vi "state.vi"(1 "buffer in":string) -> (0 "current state":dbl)   [LabVIEW 2016]
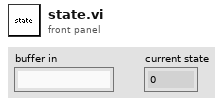
[diagram p1: front panel]
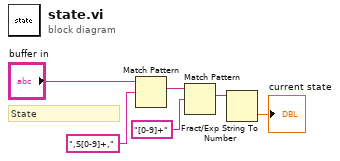
[diagram p0: block diagram]
diagram:
  # "State"
  n1 = Match Pattern(string="buffer in", regular expression=",S[0-9]+,") -> (match substring=w3:string)  [unwired: 1 in, 3 out]
  n2 = Match Pattern(string=w3, regular expression="[0-9]+") -> (match substring=w4:string)  [unwired: 1 in, 3 out]
  n3 = Fract/Exp String To Number(string=w4) -> (number=→"current state":dbl)  [unwired: 3 in, 1 out]
